vi "MetaData Parameters FG.vi"(7 "Action":T1, 8 "error in (no error)":errorcluster, 10 "MetaData Parameters":T3={"Data Type"=enum."Single Channel", "Channel Type"=enum."Format", "List"=[], "Format String"="%.3g", "Type"=enum."SGL", "Delimiter"=",", "Endian"=enum."Native"}, 11 "Item Ref in":T2 format="%.0x") -> (0 "error out":errorcluster, 2 "MetaData Parameters":T3={"Data Type"=enum."Single Channel", "Channel Type"=enum."Format", "List"=[], "Format String"="%.3g", "Type"=enum."SGL", "Delimiter"=",", "Endian"=enum."Native"}, 3 "Item Ref out":T2 format="%.0x")   [LabVIEW 2015, in "Instrument Addon Shared.lvlib"]
uses:
  Instrument Addon Shared.lvlib
  Types/MetaData Parameters.ctl
  Types/Protocol Data Type.ctl
  Types/Metadata Channel Type.ctl
  Types/Type Cast Type.ctl
  Types/Endian.ctl
  <vilib>/NI Veristand/Custom Device API/Custom Device Item Ref.ctl
  Types/FG Control.ctl
  <vilib>/NI Veristand/Custom Device API/Set Item Property (U32).vi
  <vilib>/NI Veristand/Custom Device API/Set Item Property (String).vi
  <vilib>/NI Veristand/Custom Device API/Set Item Property (String Array).vi
  <vilib>/NI Veristand/Custom Device API/Get Item Property (U32).vi
  <vilib>/NI Veristand/Custom Device API/Get Item Property (String).vi
  <vilib>/NI Veristand/Custom Device API/Get Item Property (String Array).vi
  Constants.vi
  <vilib>/NI VeriStand/Custom Device API/Custom Device API.lvlib
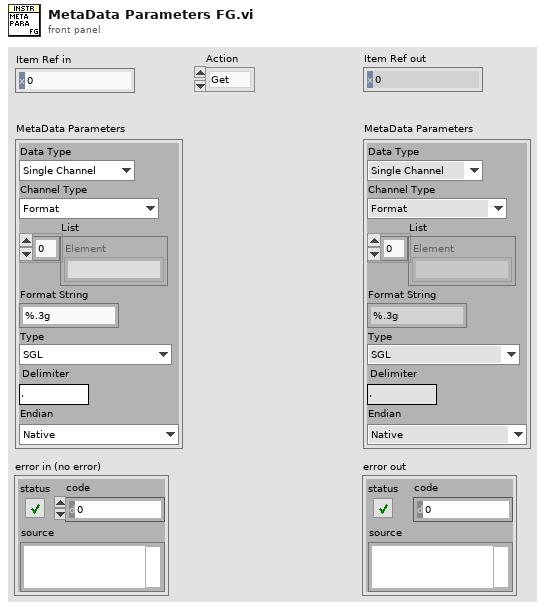
[diagram p1: front panel]
types:
  T1 = typedef "Instrument Addon Shared.lvlib/FG Control.ctl" = enum16{"Get", "Set"}
  T2 = typedef "Custom Device API.lvlib/Custom Device Item Ref.ctl" = u64
  T3 = typedef "Instrument Addon Shared.lvlib/MetaData Parameters.ctl" = cluster{"Data Type":T4, "Channel Type":T5, "List":string[], "Format String":string, "Type":T6, "Delimiter":string, "Endian":T7}
  T4 = typedef "Instrument Addon Shared.lvlib/Protocol Data Type.ctl" = enum16{"Single Channel", "Array"}
  T5 = typedef "Instrument Addon Shared.lvlib/Metadata Channel Type.ctl" = enum16{"Enumerated List", "Format", "Type Cast"}
  T6 = typedef "Instrument Addon Shared.lvlib/Type Cast Type.ctl" = enum16{"DBL", "SGL", "U64", "U32", "U16", "U8", "I64", "I32", "I16", "I8"}
  T7 = typedef "Instrument Addon Shared.lvlib/Endian.ctl" = enum16{"Native", "Little", "Big"}
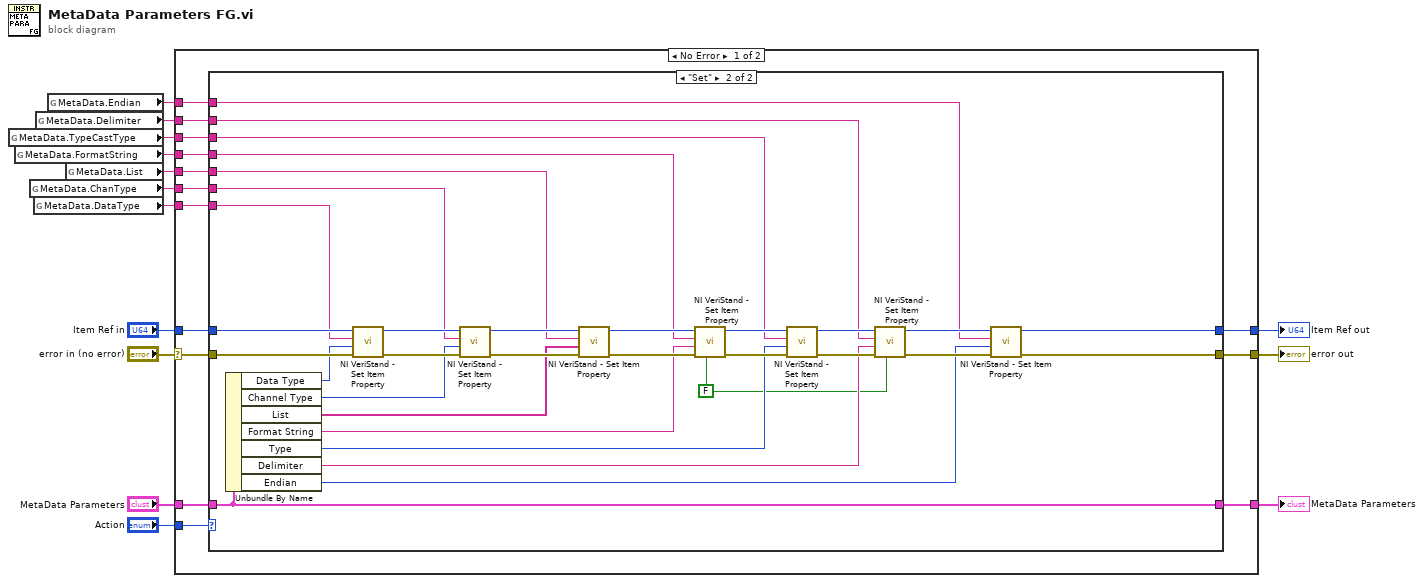
[diagram p0: block diagram]
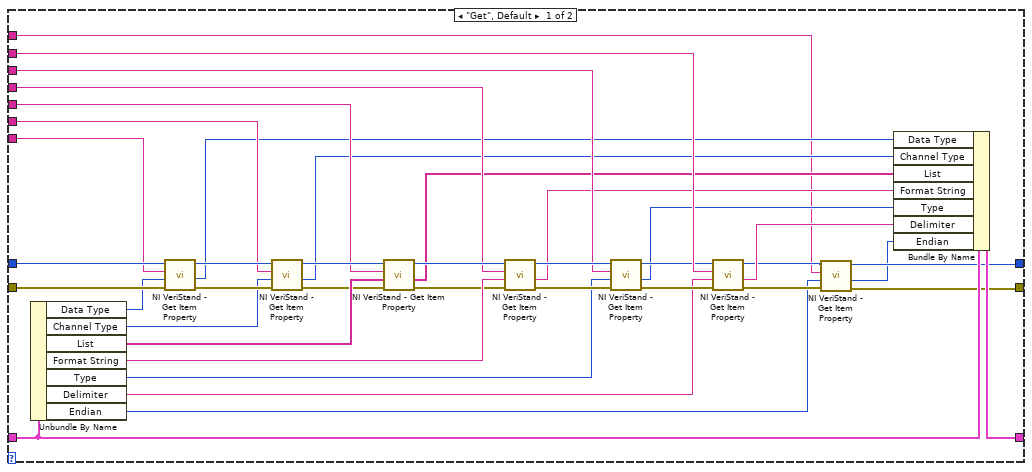
[diagram p2: hidden frame]
diagram:
  n1 = global read "Constants.vi" "MetaData.TypeCastType"() -> (w2:string)
  n2 = global read "Constants.vi" "MetaData.FormatString"() -> (w3:string)
  n3 = global read "Constants.vi" "MetaData.ChanType"() -> (w5:string)
  n4 = global read "Constants.vi" "MetaData.DataType"() -> (w6:string)
  n5 = global read "Constants.vi" "MetaData.Delimiter"() -> (w8:string)
  n6 = global read "Constants.vi" "MetaData.Endian"() -> (w1:string)
  n7 = global read "Constants.vi" "MetaData.List"() -> (w4:string)
  n8 = case shown="No Error" "error in (no error)" {
    selector: "error in (no error)" -> [w23 w102]
    tunnel: w8 -> [w28 _]
    tunnel: [w27 w100] -> w12
    tunnel: "Item Ref in" -> [w26 w100]
    tunnel: "MetaData Parameters" -> [w25 w101]
    tunnel: [w24 w102] -> w11
    tunnel: [w22 w101] -> w7
    tunnel: "Action" -> [w21 _]
    tunnel: w6 -> [w20 _]
    tunnel: w5 -> [w19 _]
    tunnel: w4 -> [w18 _]
    tunnel: w3 -> [w17 _]
    tunnel: w2 -> [w16 _]
    tunnel: w1 -> [w15 _]
    frame No Error {
      n9 = case shown="\"Set\"" w21 {
        tunnel: w28 -> [w47 w74]
        tunnel: [w34 w70] -> w27
        tunnel: w26 -> [w66 w99]
        tunnel: w25 -> [w43 w96]
        tunnel: [w32 w72] -> w24
        tunnel: w23 -> [w67 w98]
        tunnel: [w36 w96] -> w22
        tunnel: w20 -> [w62 w97]
        tunnel: w19 -> [w61 w78]
        tunnel: w18 -> [w56 w77]
        tunnel: w17 -> [w52 w76]
        tunnel: w16 -> [w48 w75]
        tunnel: w15 -> [w31 w68]
        frame "Get", Default {
          n10 = Unbundle By Name(w43) -> ("Data Type"=w65:T4, "Channel Type"=w60:T5, "List"=w59:string[], "Format String"=w55:string, "Type"=w49:T6, "Delimiter"=w44:string, "Endian"=w30:T7)
          n11 = call-poly <vilib>:"NI VeriStand - Get Item Property.vi"("error in (no error)"=w67, "Default Value"=w65, "Property Name"=w62, "Item Ref in"=w66) -> ("error out"=w64:errorcluster, "Value"=w37:u32, "Item Ref out"=w63:T2)  [unwired: 4 in, 1 out]
          n12 = call-poly <vilib>:"NI VeriStand - Get Item Property.vi"("error in (no error)"=w64, "Default Value"=w60, "Property Name"=w61, "Item Ref in"=w63) -> ("error out"=w58:errorcluster, "Value"=w38:u32, "Item Ref out"=w57:T2)  [unwired: 4 in, 1 out]
          n13 = call-poly <vilib>:"NI VeriStand - Get Item Property.vi"("error in (no error)"=w58, "Default Value"=w59, "Property Name"=w56, "Item Ref in"=w57) -> ("error out"=w54:errorcluster, "Value"=w39:string[], "Item Ref out"=w53:T2)  [unwired: 4 in, 1 out]
          n14 = call-poly <vilib>:"NI VeriStand - Get Item Property.vi"("error in (no error)"=w54, "Default Value"=w55, "Property Name"=w52, "Item Ref in"=w53) -> ("error out"=w51:errorcluster, "Value"=w40:string, "Item Ref out"=w50:T2)  [unwired: 4 in, 1 out]
          n15 = call-poly <vilib>:"NI VeriStand - Get Item Property.vi"("error in (no error)"=w51, "Default Value"=w49, "Property Name"=w48, "Item Ref in"=w50) -> ("error out"=w45:errorcluster, "Value"=w41:u32, "Item Ref out"=w46:T2)  [unwired: 4 in, 1 out]
          n16 = call-poly <vilib>:"NI VeriStand - Get Item Property.vi"("error in (no error)"=w45, "Default Value"=w44, "Property Name"=w47, "Item Ref in"=w46) -> ("error out"=w33:errorcluster, "Value"=w42:string, "Item Ref out"=w35:T2)  [unwired: 4 in, 1 out]
          n17 = call-poly <vilib>:"NI VeriStand - Get Item Property.vi"("error in (no error)"=w33, "Default Value"=w30, "Property Name"=w31, "Item Ref in"=w35) -> ("error out"=w32:errorcluster, "Value"=w29:u32, "Item Ref out"=w34:T2)  [unwired: 4 in, 1 out]
          n18 = Bundle By Name(cluster=w43, "Data Type"=w37, "Channel Type"=w38, "List"=w39, "Format String"=w40, "Type"=w41, "Delimiter"=w42, "Endian"=w29) -> (w36:T3)
        }
        frame "Set" {
          w79 = FALSE ("Binary String (T)")
          n19 = Unbundle By Name(w96) -> ("Data Type"=w95:T4, "Channel Type"=w84:T5, "List"=w83:string[], "Format String"=w82:string, "Type"=w81:T6, "Delimiter"=w80:string, "Endian"=w69:T7)
          n20 = call-poly <vilib>:"NI VeriStand - Set Item Property.vi"("error in (no error)"=w98, "Value"=w95, "Property Name"=w97, "Item Ref in"=w99) -> ("error out"=w85:errorcluster, "Item Ref out"=w94:T2)  [unwired: 5 in, 1 out]
          n21 = call-poly <vilib>:"NI VeriStand - Set Item Property.vi"("error in (no error)"=w85, "Value"=w84, "Property Name"=w78, "Item Ref in"=w94) -> ("error out"=w86:errorcluster, "Item Ref out"=w93:T2)  [unwired: 5 in, 1 out]
          n22 = call-poly <vilib>:"NI VeriStand - Set Item Property.vi"("error in (no error)"=w86, "Value"=w83, "Property Name"=w77, "Item Ref in"=w93) -> ("error out"=w87:errorcluster, "Item Ref out"=w92:T2)  [unwired: 5 in, 1 out]
          n23 = call-poly <vilib>:"NI VeriStand - Set Item Property.vi"("Binary String (T)"=w79, "error in (no error)"=w87, "Value"=w82, "Property Name"=w76, "Item Ref in"=w92) -> ("error out"=w88:errorcluster, "Item Ref out"=w91:T2)  [unwired: 4 in, 1 out]
          n24 = call-poly <vilib>:"NI VeriStand - Set Item Property.vi"("error in (no error)"=w88, "Value"=w81, "Property Name"=w75, "Item Ref in"=w91) -> ("error out"=w89:errorcluster, "Item Ref out"=w90:T2)  [unwired: 5 in, 1 out]
          n25 = call-poly <vilib>:"NI VeriStand - Set Item Property.vi"("Binary String (T)"=w79, "error in (no error)"=w89, "Value"=w80, "Property Name"=w74, "Item Ref in"=w90) -> ("error out"=w73:errorcluster, "Item Ref out"=w71:T2)  [unwired: 4 in, 1 out]
          n26 = call-poly <vilib>:"NI VeriStand - Set Item Property.vi"("error in (no error)"=w73, "Value"=w69, "Property Name"=w68, "Item Ref in"=w71) -> ("error out"=w72:errorcluster, "Item Ref out"=w70:T2)  [unwired: 5 in, 1 out]
        }
      }
    }
    frame Error {
    }
  }
  "error out" <- w11
  "MetaData Parameters" <- w7
  "Item Ref out" <- w12
